vi "Create Polynomial From Roots.vi"   [LabVIEW 2020, in "NI_AALPro.lvlib"]
doc: "Creates polynomial <B>P(x)</B> from its roots. Wire data to the <B>Roots</B> input to determine the polymorphic instance to use or manually select the instance."
uses:
  <vilib>/Analysis/NI_AALPro.lvlib
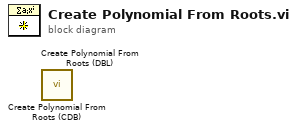
[diagram p0: block diagram]
diagram:
  n1 = call <vilib>:"Create Polynomial From Roots (CDB).vi"() -> ()  [unwired: 10 in, 2 out]
  n2 = call <vilib>:"Create Polynomial From Roots (DBL).vi"() -> ()  [unwired: 10 in, 2 out]
